vi "Main Screen.vi"() -> ()   [LabVIEW 2014]
uses:
  Controls/DataState.ctl
panel:
  out "error out":errorcluster
  in  "string":string="200000"
  in  "STOP":bool
  in  "START":bool
  in  "Exit":bool
  in  "error in (no error)":errorcluster
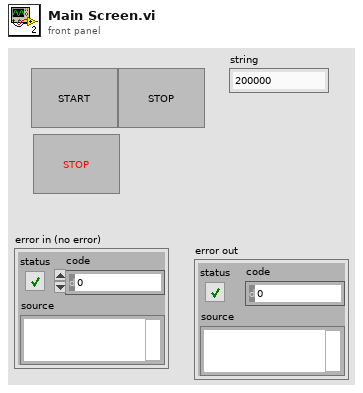
[diagram p1: front panel]
types:
  T1 = typedef "DataState.ctl" = cluster{"State":string, "Datas":variant}
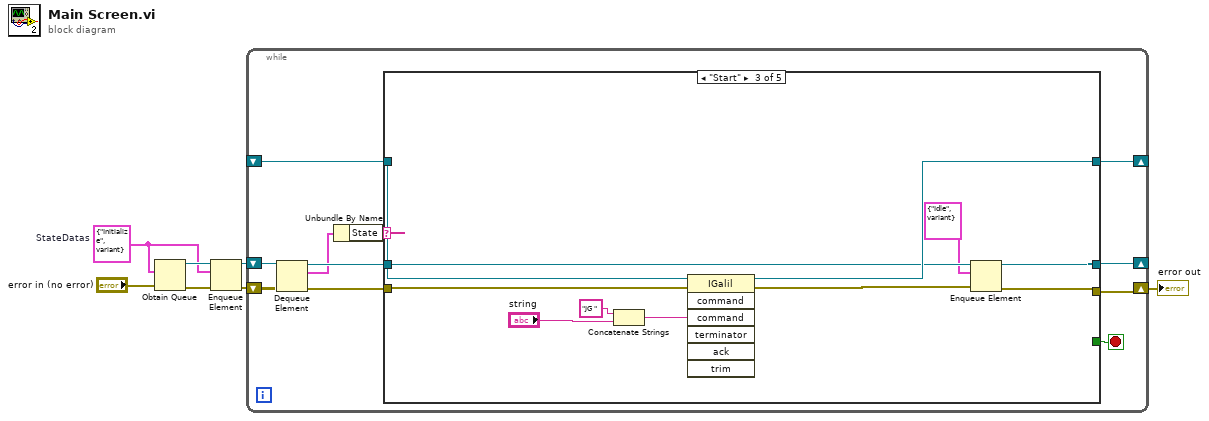
[diagram p0: block diagram]
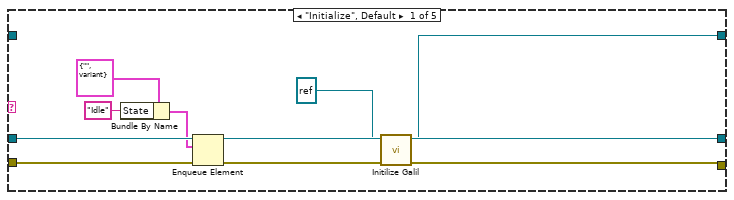
[diagram p2: hidden frame]
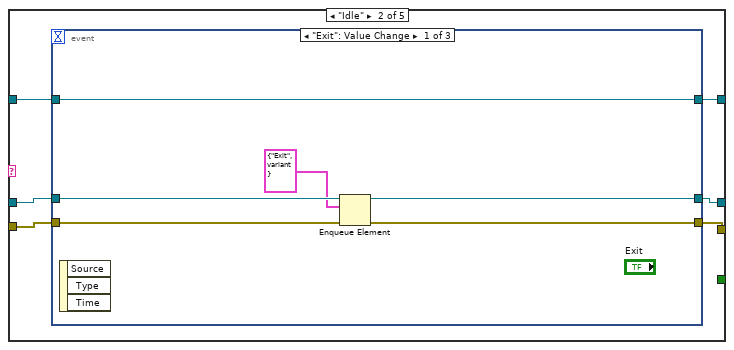
[diagram p3: hidden frame]
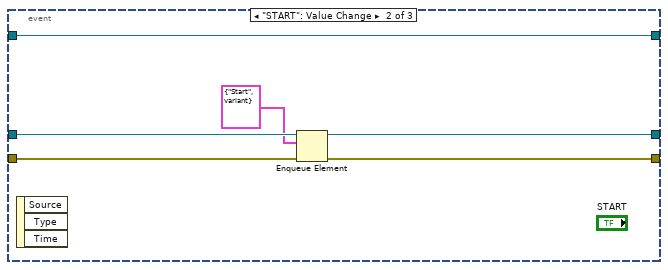
[diagram p4: hidden frame]
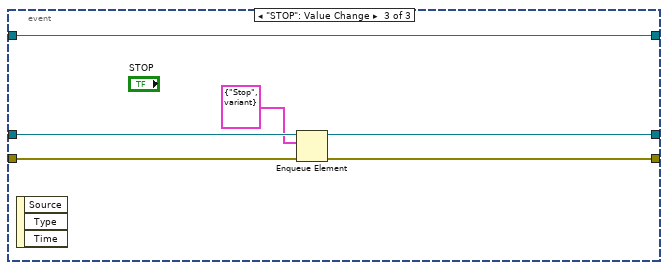
[diagram p5: hidden frame]
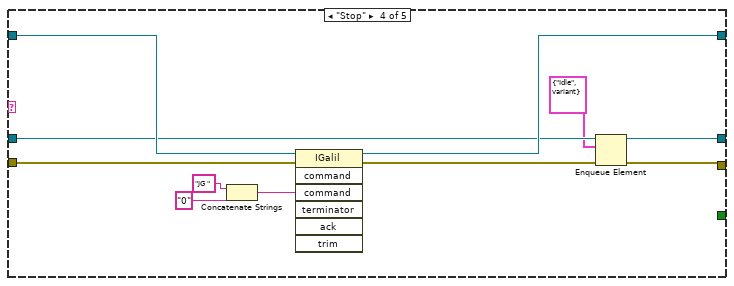
[diagram p6: hidden frame]
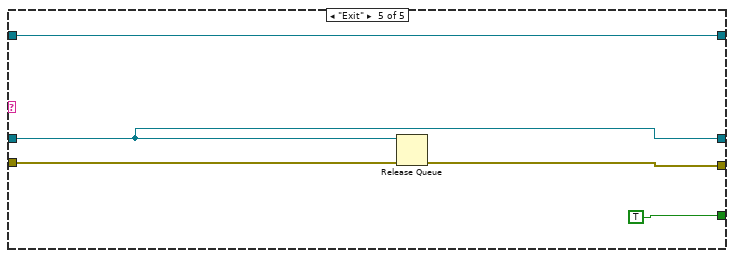
[diagram p7: hidden frame]
diagram:
  w5 = T1 {"State"="Initialize", "Datas"=variant}  # StateDatas
  n1 = Obtain Queue(element data type=w5, error in (no error)="error in (no error)") -> (queue out=w6:refnum<queue>, error out=w7:errorcluster)  [unwired: 3 in, 1 out]
  n2 = Enqueue Element(queue=w6, element=w5, error in (no error)=w7) -> (queue out=w4:refnum<queue>, error out=w2:errorcluster)  [unwired: 1 in, 1 out]
  n3 = while {
    shift-right: [w18] -> _
    shift-left: w4 -> [w17]
    shift-right: [w14] -> w1
    shift-left: w2 -> [w15]
    shift-right: [w9] -> _
    shift-left: _ -> [w8]
    stop <- w10 stop-if-true
    n4 = Dequeue Element(queue=w17, error in (no error)=w15) -> (queue out=w16:refnum<queue>, element=w12:T1, error out=w13:errorcluster)  [unwired: 1 in, 1 out]
    n5 = Unbundle By Name(w12) -> ("State"=w11:string)
    n6 = case shown="\"Start\"" w11 {
      tunnel: [w27 w34 w60 w71 w77] -> w18
      tunnel: w16 -> [w28 w33 w61 w72 w77]
      tunnel: [w20 w31 w59 w70 w78] -> w14
      tunnel: w13 -> [w26 w32 w54 w65 w79]
      tunnel: [_ _ _ _ TRUE] -> w10
      tunnel: [w19 w30 w62 w73 w75] -> w9
      tunnel: w8 -> [_ w29 w63 w74 w75]
      frame "Initialize", Default {
        n7 = Bundle By Name(cluster=T1 {"State"="", "Datas"=variant} ("element"), "State"="Idle") -> (w24:T1)
        n8 = Enqueue Element(queue=w28, element=w24, error in (no error)=w26) -> (queue out=w27:refnum<queue>, error out=w21:errorcluster)  [unwired: 1 in, 1 out]
        n9 = call "Initilize Galil.vi"("error in (no error)"=w21, "Automation Refnum in"=refnum<k7> refnum) -> ("error out"=w20:errorcluster, "Automation Refnum out"=w19:refnum<k7>)  [unwired: 7 in, 1 out]
      }
      frame "Idle" {
        n10 = event shown="[0] \"Exit\": Value Change" {
          selector: _ -> [_ _ _]
          dyn-events: _ -> [_ _ _]
          timeout: _ -> [_ _ _]
          tunnel: [w39 w45 w51] -> w34
          tunnel: w33 -> [w40 w46 w52]
          tunnel: w32 -> [w38 w44 w50]
          tunnel: [w37 w43 w49] -> w31
          tunnel: [w35 w41 w47] -> w30
          tunnel: w29 -> [w35 w41 w47]
          event "Exit": Value Change {
            n11 = event-data() -> ()  [unwired: 1 in, 3 out]
            n12 = Enqueue Element(queue=w40, element=T1 {"State"="Exit", "Datas"=variant}, error in (no error)=w38) -> (queue out=w39:refnum<queue>, error out=w37:errorcluster)  [unwired: 1 in, 1 out]
          }
          event "START": Value Change {
            n13 = event-data() -> ()  [unwired: 1 in, 3 out]
            n14 = Enqueue Element(queue=w46, element=T1 {"State"="Start", "Datas"=variant}, error in (no error)=w44) -> (queue out=w45:refnum<queue>, error out=w43:errorcluster)  [unwired: 1 in, 1 out]
          }
          event "STOP": Value Change {
            n15 = event-data() -> ()  [unwired: 1 in, 3 out]
            n16 = Enqueue Element(queue=w52, element=T1 {"State"="Stop", "Datas"=variant}, error in (no error)=w50) -> (queue out=w51:refnum<queue>, error out=w49:errorcluster)  [unwired: 1 in, 1 out]
          }
        }
      }
      frame "Start" {
        n17 = Concatenate Strings("JG " ("string"), "string") -> (w56:string)
        n18 = invoke class="IGalil" method="command"(reference=w63, error in=w54, "command"=w56) -> (reference out=w62:refnum<k7>, error out=w53:errorcluster)  [unwired: 4 in, 5 out]
        n19 = Enqueue Element(queue=w61, element=T1 {"State"="Idle", "Datas"=variant}, error in (no error)=w53) -> (queue out=w60:refnum<queue>, error out=w59:errorcluster)  [unwired: 1 in, 1 out]
      }
      frame "Stop" {
        n20 = Concatenate Strings("JG " ("string"), "0" ("string")) -> (w67:string)
        n21 = invoke class="IGalil" method="command"(reference=w74, error in=w65, "command"=w67) -> (reference out=w73:refnum<k7>, error out=w64:errorcluster)  [unwired: 4 in, 5 out]
        n22 = Enqueue Element(queue=w72, element=T1 {"State"="Idle", "Datas"=variant}, error in (no error)=w64) -> (queue out=w71:refnum<queue>, error out=w70:errorcluster)  [unwired: 1 in, 1 out]
      }
      frame "Exit" {
        n23 = Release Queue(queue=w77, error in (no error)=w79) -> (error out=w78:errorcluster)  [unwired: 1 in, 2 out]
      }
    }
  }
  "error out" <- w1
